vi "Set Macro.vi"   [LabVIEW 2016, in "Hardware.lvlib" / "Motions.lvlib" / "Motions.lvclass"]
uses:
  <userlib>/Common Components/Hardware/Abstract System/Motions/Motions/Motions.lvclass
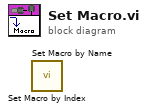
[diagram p0: block diagram]
diagram:
  n1 = call <userlib>:"Set Macro by Name.vi"() -> ()  [unwired: 9 in, 3 out]
  n2 = call <userlib>:"Set Macro by Index.vi"() -> ()  [unwired: 9 in, 3 out]
